vi "Read Source-meter.vi"(8 "error in (no error)":errorcluster, 11 "Keithley Driver in":refnum<class "Keithley Driver.lvclass">) -> (0 "error out":errorcluster, 2 "Source-meter":bool, 3 "Keithley Driver out":refnum<class "Keithley Driver.lvclass">)   [LabVIEW 2018, in "Keithley Driver.lvclass"]
uses:
  Keithley Driver.lvclass
  Keithley Driver.lvclass/Keithley Driver.ctl
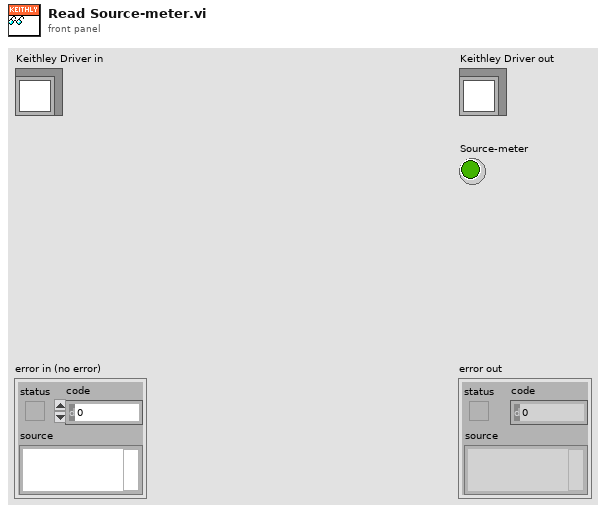
[diagram p1: front panel]
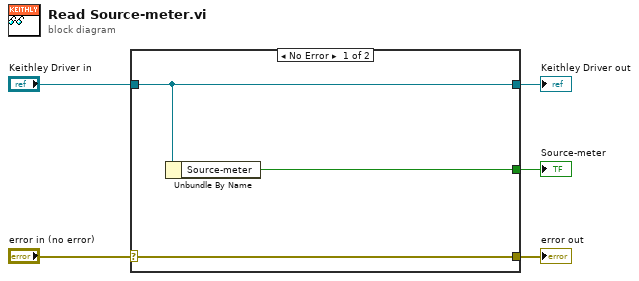
[diagram p0: block diagram]
diagram:
  n1 = case shown="No Error" "error in (no error)" {
    selector: "error in (no error)" -> [w8 w9]
    tunnel: [w8 w9] -> w4
    tunnel: [w7 w10] -> w2
    tunnel: "Keithley Driver in" -> [w7 w10]
    tunnel: [w6 _] -> w1
    frame No Error {
      n2 = Unbundle By Name(w7) -> ("Source-meter"=w6:bool)
    }
    frame Error {
    }
  }
  "error out" <- w4
  "Keithley Driver out" <- w2
  "Source-meter" <- w1
